vi "2 GV.vi"() -> ()   [LabVIEW 2020]
uses:
  <vilib>/Utility/NIReport.llb/NI_ReportGenerationCore.lvlib
  <vilib>/printing/ReportDocExtensions.llb/Append VI Block Diagram to Report (path).vi
panel:
  out "number de (0 to 1)":dbl
  out "i":dbl
  in  "Contro de interacion":dbl
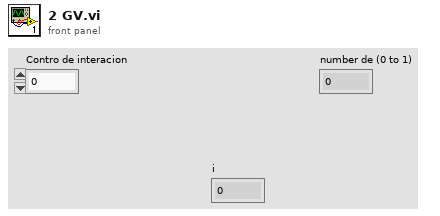
[diagram p1: front panel]
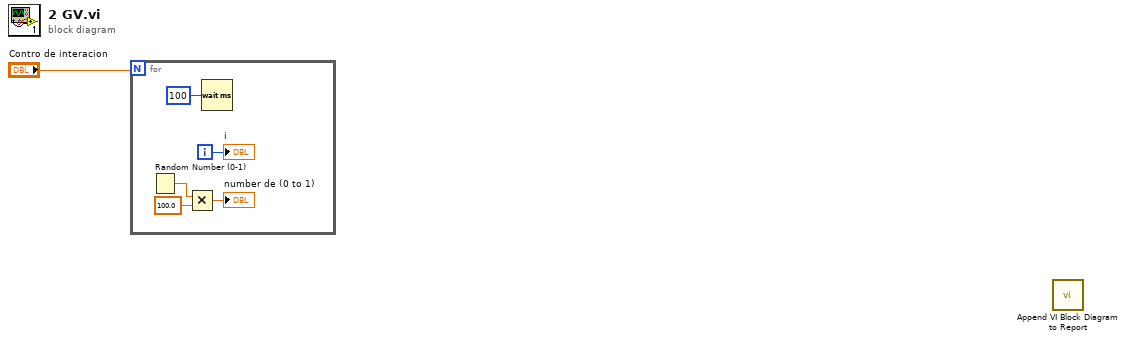
[diagram p0: block diagram]
diagram:
  n1 = for {
    N: "Contro de interacion" -> [_]
    i -> [w6]
    n2 = Random Number (0-1)() -> (number: 0 to 1=w2:dbl)
    n3 = Multiply(x=w2, y=100.0) -> (x*y=→"number de (0 to 1)":dbl)
    n4 = Wait (ms)(milliseconds to wait=100) -> ()  [unwired: 1 out]
    "i" <- w6
  }
  n5 = call-poly <vilib>:"Append VI Block Diagram to Report.vi"() -> ()  [unwired: 11 in, 5 out]
